vi "Head String[].vi"(7 "Option":T1, 8 "error in (no error)":errorcluster caption="错误输入（无错误）", 9 "ColHdrs[] Out":string[](array[string]), 10 "RowHdrs[] In":string[](array[string]), 11 "Tree Class 输入":refnum<class "Tree Class.lvclass"> caption="DNL_LabVIEW Object in") -> (0 "error out":errorcluster caption="错误输出", 1 "ColHdrS[] out":string[](array[string]), 2 "RowHdrs[] Out":string[](array[string]), 3 "Tree Class 输出":refnum<class "Tree Class.lvclass"> caption="DNL_LabVIEW Object out")   [LabVIEW 2012, in "Tree Tools.lvlib" / "Tree Class.lvclass"]
uses:
  Tree Class.lvclass
  Set Or Get Option.ctl
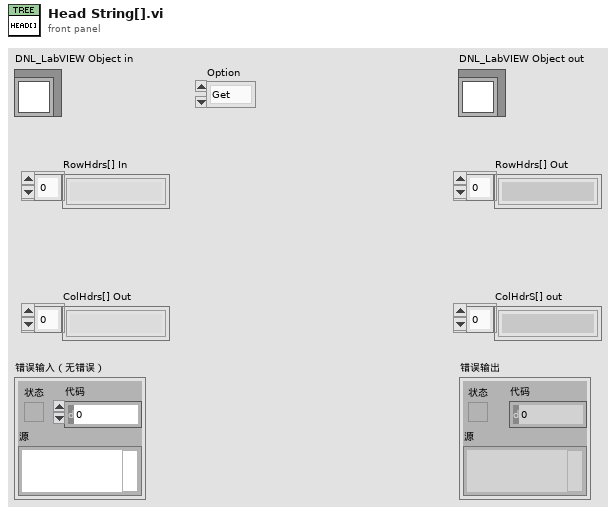
[diagram p1: front panel]
types:
  T1 = typedef "Tree Tools.lvlib/Tree Class.lvclass/Set Or Get Option.ctl" = enum16{"Get", "Set"}
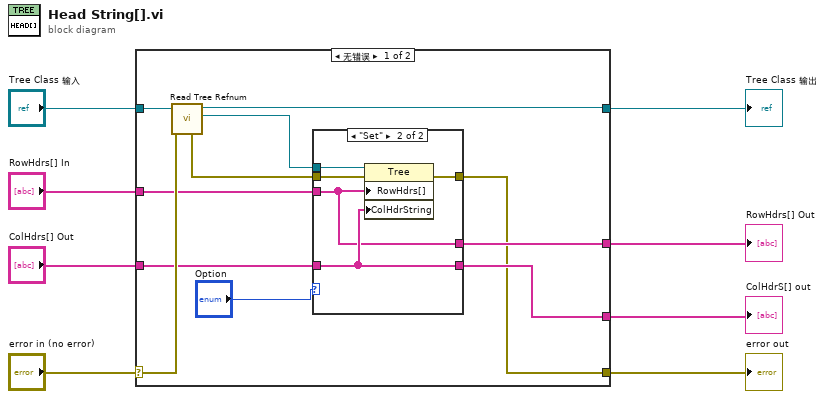
[diagram p0: block diagram]
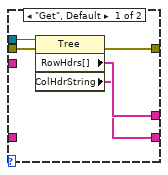
[diagram p2: hidden frame]
diagram:
  n1 = case shown="无错误" "error in (no error)" {
    selector: "error in (no error)" -> [w17 w31]
    tunnel: [w12 w31] -> w7
    tunnel: [w18 w30] -> w5
    tunnel: "Tree Class 输入" -> [w19 w30]
    tunnel: [w14 _] -> w4
    tunnel: [w13 _] -> w3
    tunnel: "RowHdrs[] In" -> [w10 _]
    tunnel: "ColHdrs[] Out" -> [w9 _]
    frame No Error {
      n2 = call-dynamic "Read Tree Refnum.vi"("error in (no error)"=w17, "Tree_LVOOP__lava_lib_tree_class in"=w19) -> ("error out"=w16:errorcluster, "Tree Refnum"=w15:refnum<vi>, "Tree_LVOOP__lava_lib_tree_class out"=w18:refnum<class "Tree Class.lvclass">)  [unwired: 7 in]
      n3 = case shown="\"Set\"" "Option" {
        tunnel: w16 -> [w24 w26]
        tunnel: w15 -> [w23 w27]
        tunnel: [w22 w28] -> w14
        tunnel: [w21 w29] -> w13
        tunnel: [w20 w25] -> w12
        tunnel: w10 -> [_ w28]
        tunnel: w9 -> [_ w29]
        frame "Get", Default {
          n4 = property class="Tree"(reference=w23, error in=w24) -> (error out=w20:errorcluster, "RowHdrs[]"=w22:string[], "ColHdrString"=w21:string[])  [unwired: 1 out]
        }
        frame "Set" {
          n5 = property class="Tree"(reference=w27, error in=w26, "RowHdrs[]"=w28, "ColHdrString"=w29) -> (error out=w25:errorcluster)  [unwired: 1 out]
        }
      }
    }
    frame Error {
    }
  }
  "error out" <- w7
  "Tree Class 输出" <- w5
  "RowHdrs[] Out" <- w4
  "ColHdrS[] out" <- w3
